vi "tcp_客户端_接收.vi"(0 "IP地址":string="127.0.0.1" caption="对方公网访问地址", 1 "端口号":i32=6314, 2 "储存路径":path=path "D:/AA") -> ()   [LabVIEW 2016, in "TCP文件传输系统.lvlib" / "TCP接收文件.lvlib"]
panel:
  out "运行中":bool
  out "单包大小":i32
  in  "分一包（兆）":i64=40
  out "已收百分比":string
  out "帧数":i32
  out "帧号":i32
  out "生成新的保存路径":path
  out "需接收次数":i32
  out "文件名":string
  out "已收次数":i32
  out "error out":errorcluster
  out "当前步骤":T1(ring)
  out "错误输出":errorcluster
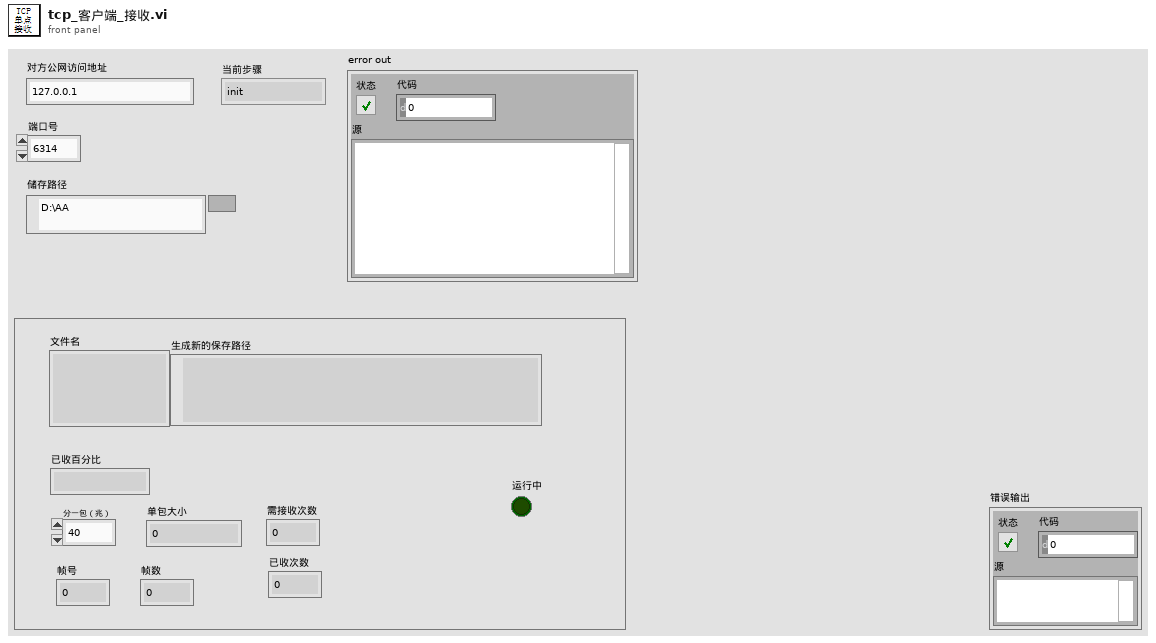
[diagram p1: front panel]
types:
  T1 = enum16{"init", "receivehead", "receivecontent", "receivesuccess", "over"}
  T2 = enum16{"open", "replace", "create", "open or create", "replace or create", "replace or create with confirmation"}
  T3 = cluster{"网络灯":bool, "接收中":bool, "已接收百分比":u8, "接收成功次数":dbl}
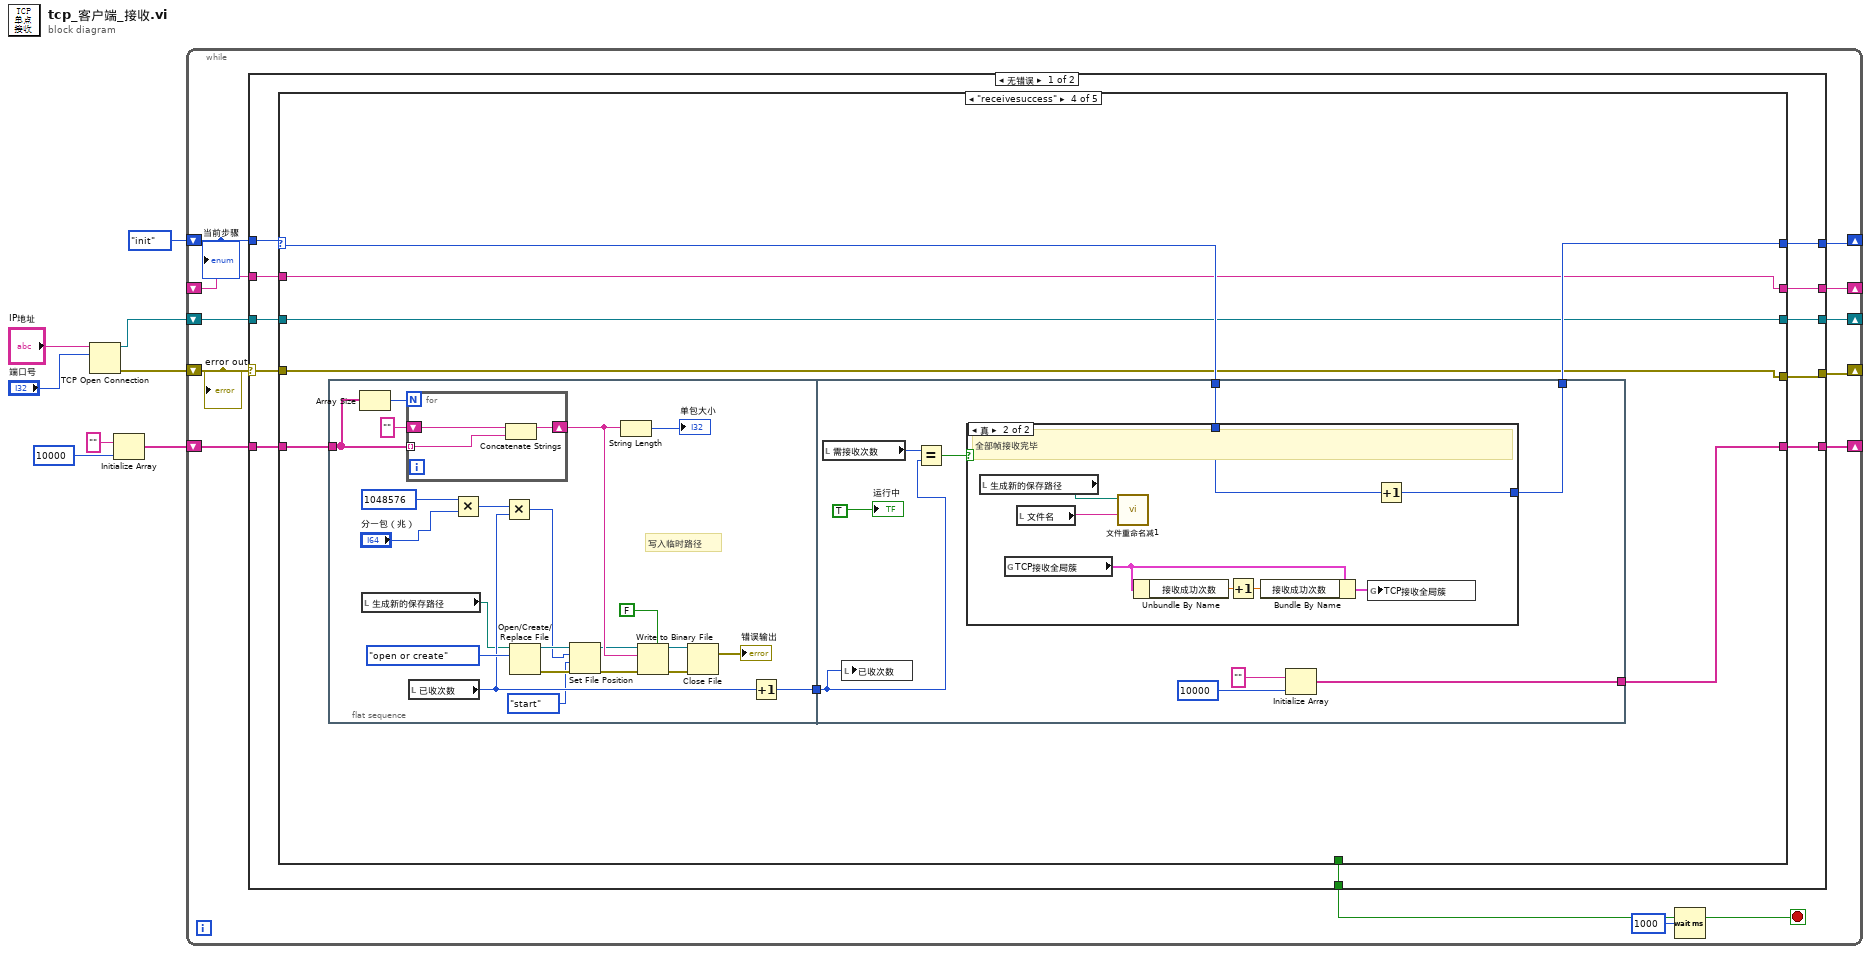
[diagram p0: block diagram]
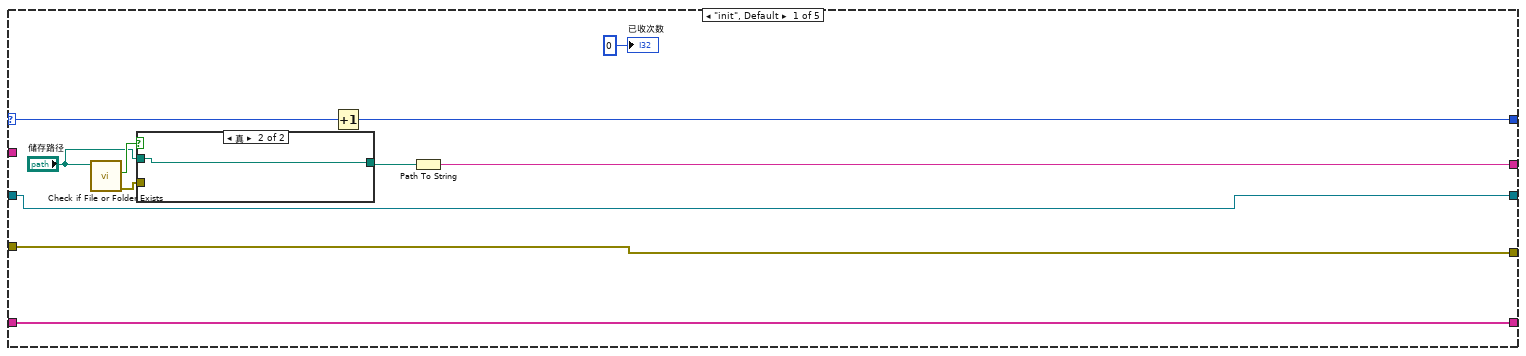
[diagram p2: hidden frame]
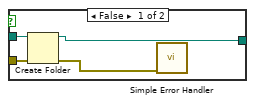
[diagram p3: hidden frame]
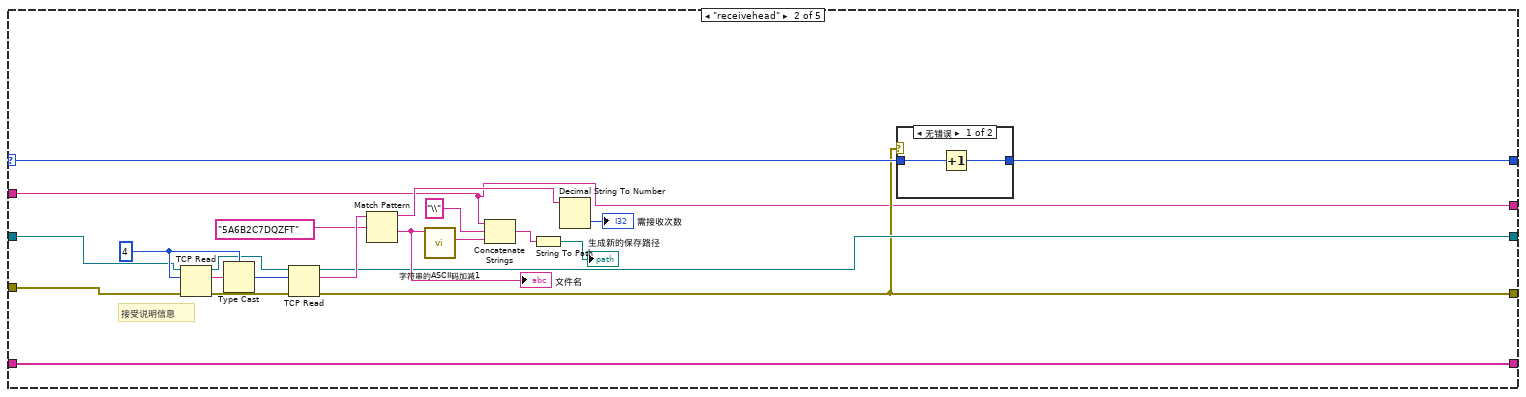
[diagram p4: hidden frame]
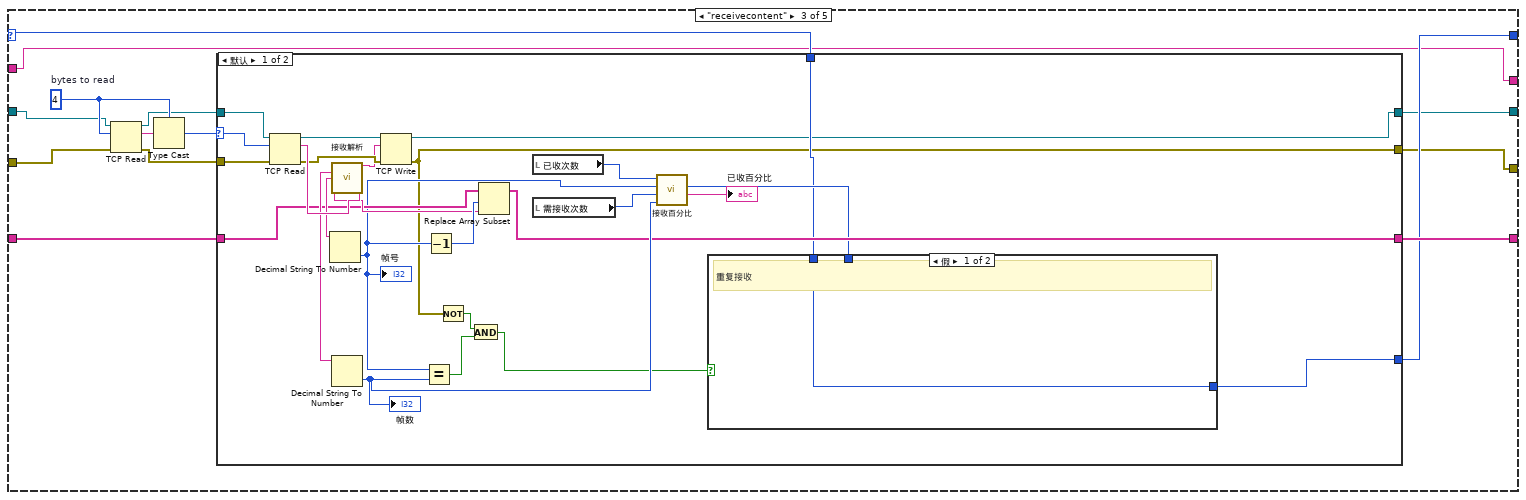
[diagram p6: hidden frame]
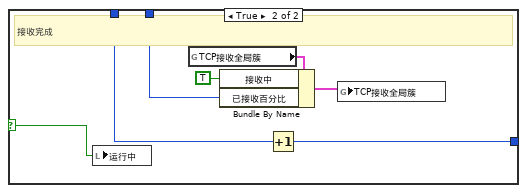
[diagram p7: hidden frame]
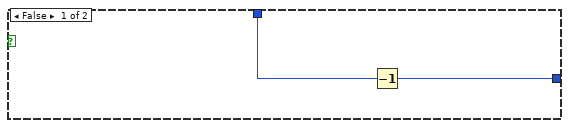
[diagram p9: hidden frame]
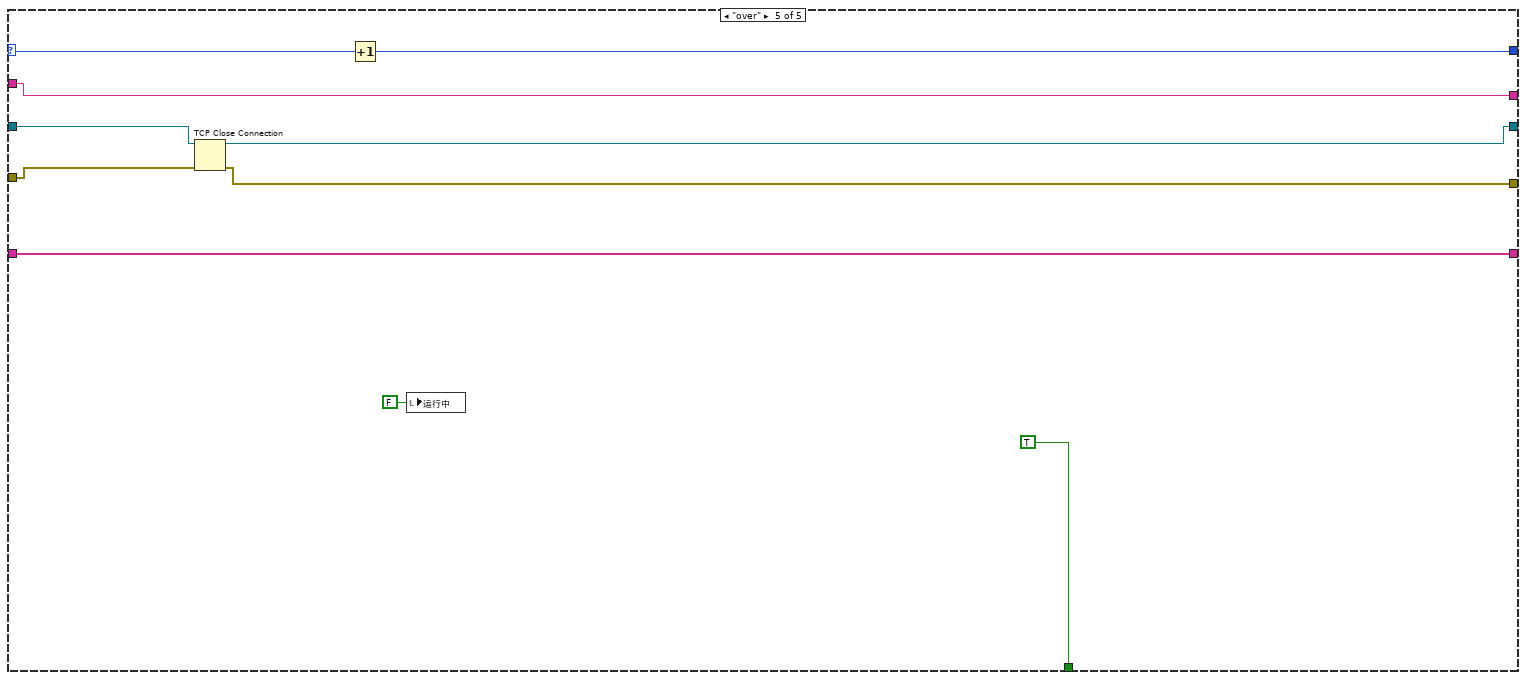
[diagram p10: hidden frame]
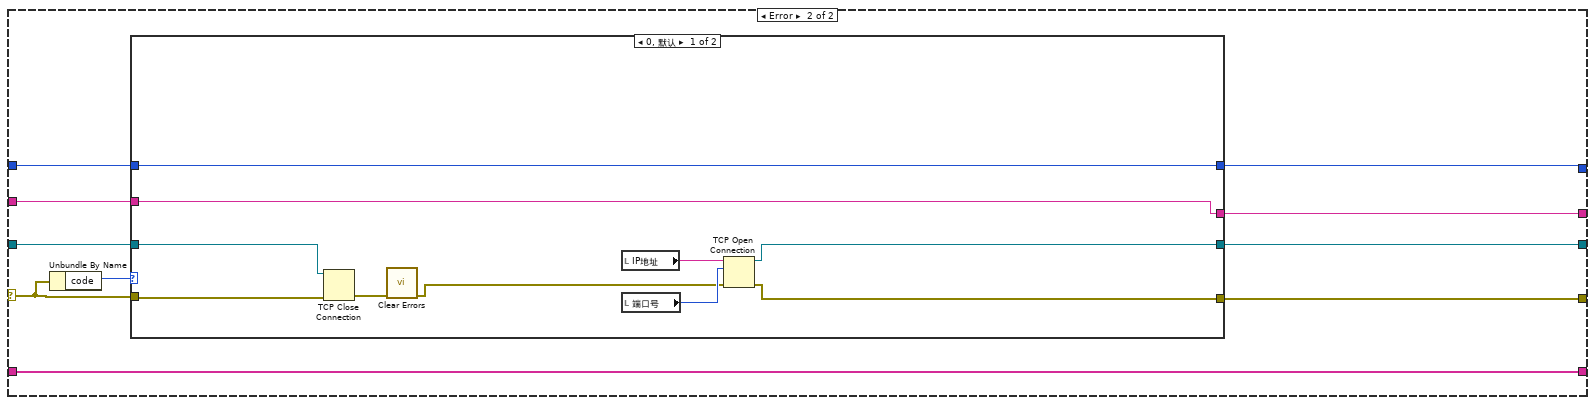
[diagram p11: hidden frame]
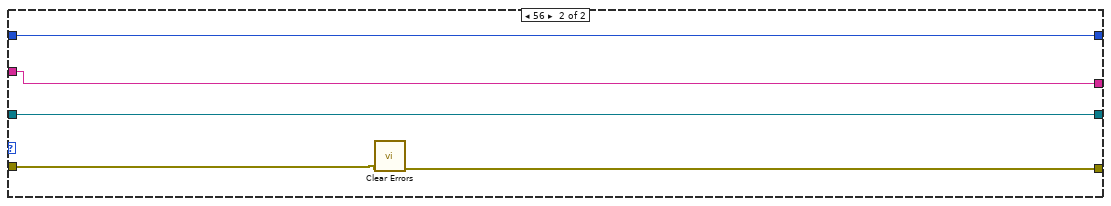
[diagram p12: hidden frame]
diagram:
  n1 = TCP Open Connection(address="IP地址", remote port or service name="端口号") -> (connection ID=w2:refnum<k5>, error out=w3:errorcluster)  [unwired: 3 in]
  n2 = Initialize Array("", 10000 ("维数大小")) -> (w1:string[])
  n3 = while {
    shift-right: [w19] -> _
    shift-left: T1."init" -> [w20]
    shift-right: [w15] -> _
    shift-left: w3 -> [w16]
    shift-right: [w13] -> _
    shift-left: w2 -> [w14]
    shift-right: [w12] -> _
    shift-left: _ -> [w11]
    shift-right: [w9] -> _
    shift-left: w1 -> [w10]
    stop <- w18 stop-if-true
    n4 = case shown="无错误" w16 {
      selector: w16 -> [w26 w195]
      tunnel: w20 -> [w31 w191]
      tunnel: [w30 w190] -> w19
      tunnel: [w29 _] -> w18
      tunnel: [w24 w194] -> w15
      tunnel: w14 -> [w27 w193]
      tunnel: [w23 w192] -> w13
      tunnel: [w28 w188] -> w12
      tunnel: w11 -> [w25 w189]
      tunnel: w10 -> [w22 w187]
      tunnel: [w21 w187] -> w9
      frame No Error {
        n5 = case shown="\"receivesuccess\"" w31 {
          selector: w31 -> [w42 w69 w77 w128 w186]
          tunnel: [w41 w68 w76 w129 w185] -> w30
          tunnel: [_ _ _ _ TRUE] -> w29
          tunnel: [w35 w49 w73 w125 w177] -> w28
          tunnel: w27 -> [w34 w60 w83 w126 w182]
          tunnel: w26 -> [w33 w59 w84 w127 w181]
          tunnel: w25 -> [_ w49 w73 w125 w177]
          tunnel: [w33 w50 w75 w127 w179] -> w24
          tunnel: [w34 w51 w74 w126 w180] -> w23
          tunnel: w22 -> [w32 w48 w81 w131 w178]
          tunnel: [w32 w48 w78 w130 w178] -> w21
          frame "init", Default {
            n6 = call <vilib>:"Check if File or Folder Exists.vi"("path"="储存路径") -> ("error out"=w38:errorcluster, "file or folder exists?"=w39:bool)  [unwired: 8 in, 1 out]
            n7 = case shown="真" w39 {
              tunnel: "储存路径" -> [w46 w47]
              tunnel: w38 -> [w45 _]
              tunnel: [w44 w47] -> w36
              frame False {
                n8 = Create Folder(path (use dialog)=w46, error in=w45) -> (created path=w44:path, error out=w43:errorcluster)  [unwired: 1 in, 1 out]
                n9 = call <vilib>:"Simple Error Handler.vi"("error in (no error)"=w43) -> ()  [unwired: 4 in, 5 out]
              }
              frame True {
              }
            }
            n10 = Increment(x=w42) -> (x+1=w41:T1)
            n11 = Path To String(path=w36) -> (string=w35:string)
            "已收次数" <- i64 0 ("已发次数")
          }
          frame "receivehead" {
            w67 = 4 ("读取的字节")
            # "接受说明信息"
            n12 = TCP Read(connection ID=w60, bytes to read=w67, error in (no error)=w59) -> (connection ID out=w63:refnum<k5>, data out=w66:string, error out=w64:errorcluster)  [unwired: 2 in]
            n13 = Type Cast(type=w67, x=w66) -> (*(type *) &x=w65:i32)
            n14 = TCP Read(connection ID=w63, bytes to read=w65, error in (no error)=w64) -> (connection ID out=w51:refnum<k5>, data out=w62:string, error out=w50:errorcluster)  [unwired: 2 in]
            n15 = Match Pattern(string=w62, regular expression="5A6B2C7DQZFT" ("正则表达式")) -> (before substring=w55:string, after substring=w58:string)  [unwired: 1 in, 2 out]
            "文件名" <- w58
            n16 = call "字符串的ASCII码加减1.vi"("原字符串"=w58) -> ("ASCII码"=w57:string)  [unwired: 10 in]
            n17 = Concatenate Strings(w49, "\\" ("字符串"), w57) -> (w52:string)
            n18 = String To Path(string=w52) -> (path=→"生成新的保存路径":path)
            n19 = Decimal String To Number(string=w55) -> (number=→"需接收次数":i32)  [unwired: 2 in, 1 out]
            n20 = case shown="无错误" w50 {
              tunnel: w69 -> [w71 w72]
              tunnel: [w70 w72] -> w68
              frame No Error {
                n21 = Increment(x=w71) -> (x+1=w70:T1)
              }
              frame Error {
              }
            }
          }
          frame "receivecontent" {
            w86 = 4  # bytes to read
            n22 = TCP Read(connection ID=w83, bytes to read=w86, error in (no error)=w84) -> (connection ID out=w80:refnum<k5>, data out=w85:string, error out=w79:errorcluster)  [unwired: 2 in]
            n23 = Type Cast(type=w86, x=w85) -> (*(type *) &x=w82:i32)
            n24 = case shown="默认" w82 {
              selector: w82 -> [w99 _]
              tunnel: w81 -> [w102 w123]
              tunnel: w80 -> [w101 w121]
              tunnel: w79 -> [w100 w122]
              tunnel: [w93 w123] -> w78
              tunnel: w77 -> [w90 w124]
              tunnel: [w89 w124] -> w76
              tunnel: [w88 w122] -> w75
              tunnel: [w87 w121] -> w74
              frame Default {
                n25 = TCP Read(connection ID=w101, bytes to read=w99, error in (no error)=w100) -> (connection ID out=w109:refnum<k5>, data out=w112:string, error out=w108:errorcluster)  [unwired: 2 in]
                n26 = call "接收解析.vi"("data in"=w112) -> ("重算CRC32"=w106:string, "帧数"=w107:string, "帧号"=w111:string, "帧内容"=w105:string)  [unwired: 3 in, 8 out]
                n27 = Decimal String To Number(string=w111) -> (number=w96:i32)  [unwired: 2 in, 1 out]
                "帧号" <- w96
                n28 = Decimal String To Number(string=w107) -> (number=w95:i32)  [unwired: 2 in, 1 out]
                "帧数" <- w95
                n29 = TCP Write(connection ID=w109, data in=w106, error in (no error)=w108) -> (connection ID out=w87:refnum<k5>, error out=w88:errorcluster)  [unwired: 1 in, 1 out]
                n30 = Equal?(x=w96, y=w95) -> (x = y?=w104:bool)
                n31 = Decrement(x=w96) -> (x-1=w110:i32)
                n32 = Not(x=w88) -> (.not. x?=w103:bool)
                n33 = And(x=w103, y=w104) -> (x .and. y?=w92:bool)
                n34 = Replace Array Subset(array=w102, new element=w105, index=w110) -> (w93:string[])
                n35 = local read "已收次数"() -> (w98:i32)
                n36 = local read "需接收次数"() -> (w97:i32)
                n37 = call "接收百分比.vi"("需发送次数"=w95, "帧数"=w97, "帧号"=w96, "已收次数"=w98) -> (1:"已收百分比"=→"已收百分比":string, 2:"已收百分比"=w91:u8)  [unwired: 6 in]
                n38 = case shown="假" w92 {
                  selector: w92 -> [_ w114]
                  tunnel: w91 -> [_ w117]
                  tunnel: w90 -> [w113 w116]
                  tunnel: [w113 w115] -> w89
                  frame False {
                    # "重复接收"
                  }
                  frame True {
                    # "接收完成"
                    n39 = local write "运行中"(w114) -> ()
                    n40 = global read "全局变量1.vi" "TCP接收全局簇"() -> (w120:T3)
                    n41 = Bundle By Name(cluster=w120, "接收中"=TRUE, "已接收百分比"=w117) -> (w119:T3)
                    n42 = Increment(x=w116) -> (x+1=w115:T1)
                    n43 = global write "全局变量1.vi" "TCP接收全局簇"(w119) -> ()
                  }
                }
              }
              frame ..0 {
                # "content为空"
              }
            }
          }
          frame "receivesuccess" {
            n44 = flat-sequence {
              tunnel: w131 -> [w146]
              tunnel: [w154] -> w132
              tunnel: w132 -> [w166]
              tunnel: [w161] -> w130
              tunnel: w128 -> [w159]
              tunnel: [w158] -> w129
              frame #0 {
                # "写入临时路径"
                n45 = Array Size(array=w146) -> (size(s)=w147:i32)
                n46 = local read "生成新的保存路径"() -> (w133:path)
                n47 = for {
                  N: w147 -> [_]
                  shift-right: [w157] -> w145
                  shift-left: "" -> [w156]
                  tunnel: w146 -> [w155] mode=indexing
                  n48 = Concatenate Strings(w156, w155) -> (w157:string)
                }
                n49 = local read "已收次数"() -> (w139:i32)
                n50 = Multiply(x=i64 1048576, y="分一包（兆）") -> (x*y=w135:i64)
                n51 = Multiply(x=w135, y=w139) -> (x*y=w138:i64)
                n52 = Open/Create/Replace File(file path (use dialog)=w133, operation (0:open)=T2."open or create" ("操作(0:open)")) -> (refnum out=w142:refnum<file>, error out=w143:errorcluster)  [unwired: 4 in, 1 out]
                n53 = Set File Position(offset (in bytes) (0)=w138, refnum=w142, from (0:start)=enum16{"start", "end", "current"}."start" ("自（0:起始）"), error in=w143) -> (refnum out=w140:refnum<file>, error out=w141:errorcluster)
                n54 = String Length(string=w145) -> (length=→"单包大小":i32)
                n55 = Write to Binary File(file (use dialog)=w140, data=w145, error in=w141, 5:FALSE ("预置数组或字符串大小？(T)")) -> (refnum out=w152:refnum<file>, error out=w153:errorcluster)  [unwired: 2 in, 1 out]
                n56 = Close File(refnum=w152, error in=w153) -> (error out=→"错误输出":errorcluster)  [unwired: 1 out]
                n57 = Increment(x=w139) -> (x+1=w154:i32)
              }
              frame #1 {
                n58 = local read "需接收次数"() -> (w165:i32)
                n59 = local write "已收次数"(w166) -> ()
                n60 = Equal?(x=w165, y=w166) -> (x = y?=w164:bool)
                n61 = case shown="真" w164 {
                  tunnel: w159 -> [w168 w170]
                  tunnel: [w167 w169] -> w158
                  frame False {
                    n62 = Decrement(x=w168) -> (x-1=w167:T1)
                  }
                  frame True {
                    # "全部帧接收完毕"
                    n63 = local read "生成新的保存路径"() -> (w176:path)
                    n64 = global read "全局变量1.vi" "TCP接收全局簇"() -> (w171:T3)
                    n65 = local read "文件名"() -> (w175:string)
                    n66 = call "文件重命名减1.vi"("名称或相对路径"=w175, "源路径"=w176) -> ()  [unwired: 10 in]
                    n67 = Unbundle By Name(w171) -> ("接收成功次数"=w172:dbl)
                    n68 = Increment(x=w172) -> (x+1=w173:dbl)
                    n69 = Bundle By Name(cluster=w171, "接收成功次数"=w173) -> (w174:T3)
                    n70 = global write "全局变量1.vi" "TCP接收全局簇"(w174) -> ()
                    n71 = Increment(x=w170) -> (x+1=w169:T1)
                  }
                }
                n72 = Initialize Array("", 10000 ("维数大小")) -> (w161:string[])
                "运行中" <- TRUE ("运行指示灯")
              }
            }
          }
          frame "over" {
            n73 = TCP Close Connection(connection ID=w182, error in (no error)=w181) -> (connection ID out=w180:refnum<k5>, error out=w179:errorcluster)  [unwired: 1 in]
            n74 = Increment(x=w186) -> (x+1=w185:T1)
            n75 = local write "运行中"(FALSE ("运行中")) -> ()
          }
        }
      }
      frame Error {
        n76 = Unbundle By Name(w195) -> ("code"=w196:i32)
        n77 = case shown="0, 默认" w196 {
          tunnel: w195 -> [w203 w211]
          tunnel: [w199 w210] -> w194
          tunnel: w193 -> [w202 w207]
          tunnel: [w200 w207] -> w192
          tunnel: w191 -> [w198 w209]
          tunnel: [w198 w209] -> w190
          tunnel: w189 -> [w197 w208]
          tunnel: [w197 w208] -> w188
          frame 0, Default {
            n78 = TCP Close Connection(connection ID=w202, error in (no error)=w203) -> (error out=w204:errorcluster)  [unwired: 1 in, 1 out]
            n79 = call <vilib>:"Clear Errors.vi"("error in (no error)"=w204) -> ("error out"=w201:errorcluster)  [unwired: 5 in, 1 out]
            n80 = local read "IP地址"() -> (w206:string)
            n81 = local read "端口号"() -> (w205:i32)
            n82 = TCP Open Connection(address=w206, remote port or service name=w205, error in (no error)=w201) -> (connection ID=w200:refnum<k5>, error out=w199:errorcluster)  [unwired: 2 in]
          }
          frame 56 {
            n83 = call <vilib>:"Clear Errors.vi"("error in (no error)"=w211) -> ("error out"=w210:errorcluster)  [unwired: 5 in, 1 out]
          }
        }
      }
    }
    n84 = Wait (ms)(milliseconds to wait=u32 1000 ("等待时间（毫秒）")) -> ()  [unwired: 1 out]
    "当前步骤" <- w20
    "error out" <- w16
  }
